vi "DM_Amplitude_Update.vi"(1 "Adaptive Astigmatism Value":dbl=1.5, 2 "Step #":u16) -> ()   [LabVIEW 2015]
panel:
  out "New Values":string[](array[string])
  out "Decimal":bool[](array[boolean])
  out "Less than or equal to":bool[](array[boolean])
  out "And":bool[](array[boolean])
  in  "Aberrations ID":string[][](array[string])=[["Flatmap 1", "1.0"], ["Flatmap 2", "0"], ["Ast (normal)", "1"], ["0", "1"], ["3", "1"], ["7", "1"], ["11", "0"], ["15", "0"]]
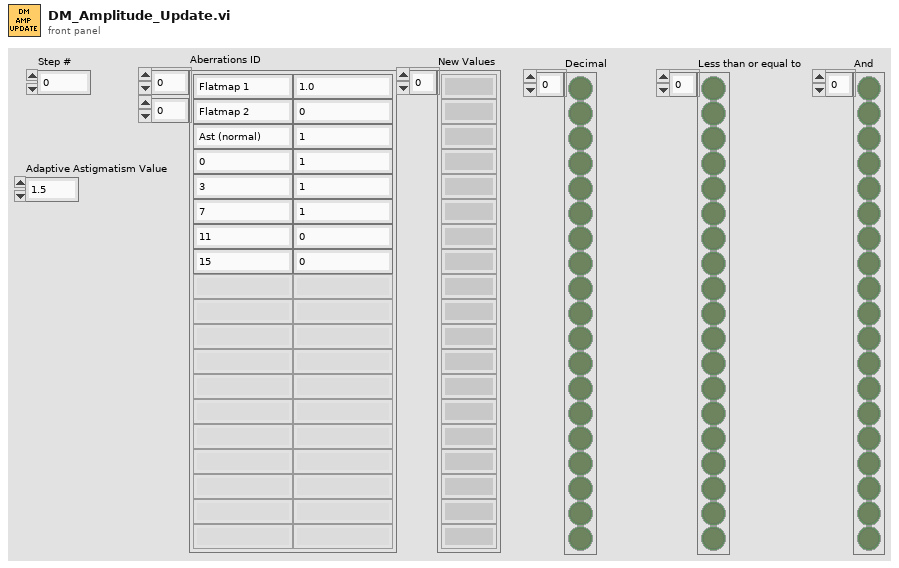
[diagram p1: front panel]
types:
  T1 = typedef "AbberationControl.ctl" = cluster{"Abberations":dbl[][], "Modes":i32[], "Flat":dbl[], "Abberations ID":string[][]}
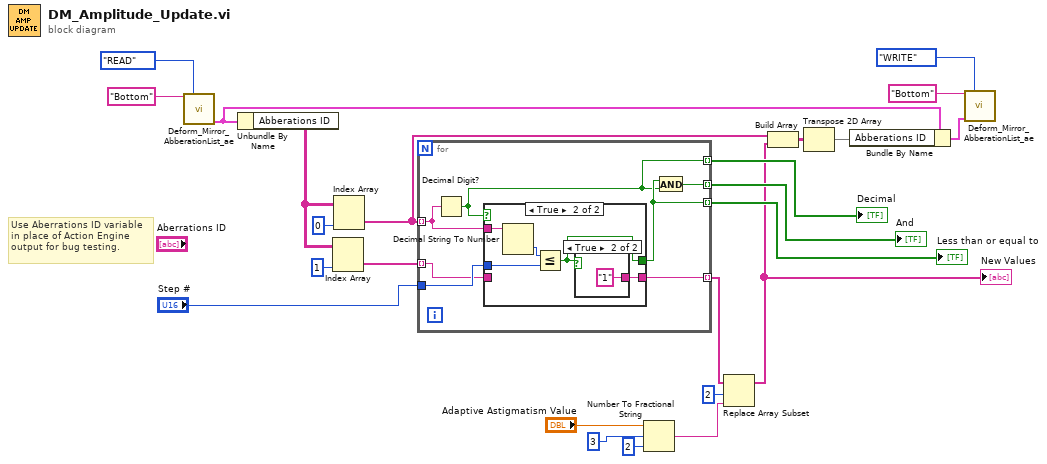
[diagram p0: block diagram]
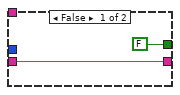
[diagram p2: hidden frame]
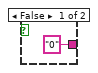
[diagram p3: hidden frame]
diagram:
  # "Use Aberrations ID variable\nin place of Action Engine \noutput for bug testing."
  n1 = call "Deform_Mirror_AbberationList_ae.vi"("Mirror ID"="Bottom", "Enum"=enum16{"WRITE", "READ"}."READ") -> ("Abberation Cluster Out"=w14:T1)  [unwired: 12 in, 1 out]
  n2 = Unbundle By Name(w14) -> ("Abberations ID"=w1:string[][])
  n3 = Index Array(array=w1, index (col)=1 ("disabled index (col)")) -> (element=w4:string[])  [unwired: 1 in]
  n4 = Index Array(array=w1, index (col)=0 ("disabled index (col)")) -> (element=w12:string[])  [unwired: 1 in]
  n5 = for {
    tunnel: w12 -> [w30] mode=indexing
    tunnel: [w31] -> w24 mode=indexing
    tunnel: [w28] -> w21 mode=indexing
    tunnel: [w25] -> w20 mode=indexing
    tunnel: "Step #" -> [w29]
    tunnel: w4 -> [w27] mode=indexing
    tunnel: [w26] -> w3 mode=indexing
    n6 = Decimal Digit?(1:w30) -> (0:w25:bool)
    n7 = case shown="True" w25 {
      tunnel: w30 -> [_ w38]
      tunnel: w29 -> [_ w37]
      tunnel: [FALSE w34] -> w28
      tunnel: w27 -> [w32 _]
      tunnel: [w32 w35] -> w26
      frame False {
      }
      frame True {
        n8 = Decimal String To Number(string=w38) -> (number=w36:i32)  [unwired: 2 in, 1 out]
        n9 = Less Or Equal?(x=w36, y=w37) -> (x <= y?=w34:bool)
        n10 = case shown="True" w34 {
          tunnel: ["0" "1"] -> w35
          frame False {
          }
          frame True {
          }
        }
      }
    }
    n11 = And(x=w28, y=w25) -> (x .and. y?=w31:bool)
  }
  "And" <- w24
  "Less than or equal to" <- w21
  "Decimal" <- w20
  n12 = Number To Fractional String(number="Adaptive Astigmatism Value", width (-)=i16 3, precision (6)=i16 2) -> (F-format string=w5:string)  [unwired: 1 in]
  n13 = Replace Array Subset(array=w3, new element=w5, index=2) -> (w2:string[])
  "New Values" <- w2
  n14 = Build Array(w12, w2) -> (w11:string[][])
  n15 = Transpose 2D Array(2D array=w11) -> (transposed array=w10:string[][])
  n16 = Bundle By Name(cluster=w14, "Abberations ID"=w10) -> (w13:T1)
  n17 = call "Deform_Mirror_AbberationList_ae.vi"("Mirror ID"="Bottom", "Enum"=enum16{"WRITE", "READ"}."WRITE", "Abberation Cluster In"=w13) -> ()  [unwired: 11 in, 2 out]
